vi "Global Constants.vi"() -> ()   [LabVIEW 2026, in "TALOS.lvlib"]
doc: "This is just a container for inner-library constant (i.e. ABORT variable actual name)."
uses:
  TALOS.lvlib
  <vilib>/Utility/miscctls.llb/LVBoundsTypeDef.ctl
panel:
  out "TCP Base Port":u16=40000
  out "Text GD Msg Separator":string=";"
  in  "uS Sub Panel Bounds":T1={"Width"=1621, "Height"=768}
  out "uSs not to close when realigning Run Config":string[](array[string])=["DAQ Sender", "GUI of", "TCP Server", "Subpanel", "TCP Listener", "TCP Writer", "Local Error Manager", "Postman"]
  out "Run config folder":string="Run configurations"
  out "uS not logging Consumer cases":string[](array[string])
  out "uS classes with Safe Mode unfiltered":string[](array[string])=["Common GUI v3", "Error Manager", "Guardian Subpanel", "Kasli Listener", "Kasli Writer", "TCP Listener", "TCP Writer", "TCP Server", "Postman", "DAQ Sender", "Local Error Manager"]
  out "TCP Timeout (ms)":i32=2000
  out "Max TCP Packet Size":i32=10000000
  out "TCP Server Port":u16=1818
  out "ABORT Crt Lvl":u8=4
  out "\"Smart\" uService":string="Tamer"
  out "GUI Class Name":string="Common GUI v3"
  in  "Local":bool
  # "These uServices produce too many Consumer cases per minutes, and they will blow up easily the System and the Personal log."
  # "In Safe Mode, responses to messages are disabled, to ensure that no uService will inadvertitedly exit the Safe Mode before time. This list comprises the Uservices that, for system reasons, still needs to properly parse incoming messages."
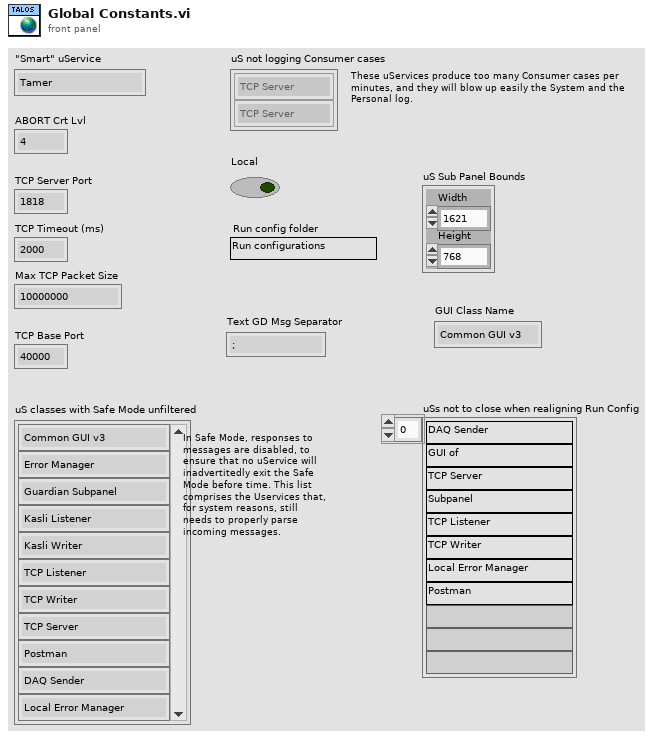
[diagram p1: front panel]
types:
  T1 = typedef "LVBoundsTypeDef.ctl" = cluster{"Width":u32, "Height":u32}
diagram:
